vi "Connect_AMI.vi"(1 "error in":T2, 2 "Communications Config":T1={"connection ID"=refnum, "IP"="111.111.111.2", "TCP Port"=7180}) -> (0 "error out":T2)   [LabVIEW 2016]
uses:
  Instrument_Setup.vi
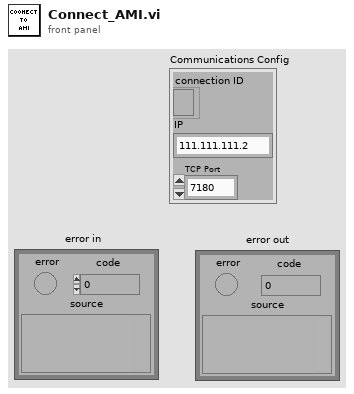
[diagram p1: front panel]
types:
  T1 = cluster{"connection ID":refnum<k5>, "IP":string, "TCP Port":i32}
  T2 = cluster{"error":bool, "code":i32, "source":string}
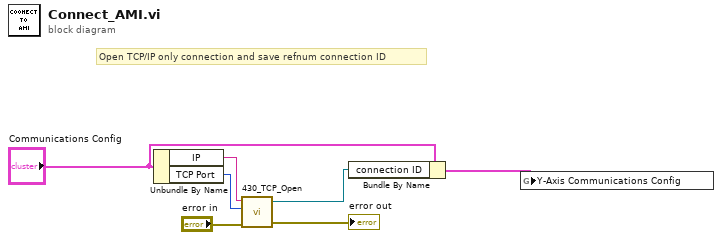
[diagram p0: block diagram]
diagram:
  # "Open TCP/IP only connection and save refnum connection ID"
  n1 = Unbundle By Name("Communications Config") -> ("IP"=w7:string, "TCP Port"=w2:i32)
  n2 = call "430_TCP_Open.vi"("IP Address"=w7, "TCP Port"=w2, "error in (no error)"="error in") -> ("connection ID"=w3:refnum<k5>, "error out"=→"error out":errorcluster)  [unwired: 3 in, 1 out]
  n3 = Bundle By Name(cluster="Communications Config", "connection ID"=w3) -> (w5:T1)
  n4 = global write "Instrument_Setup.vi" "Y-Axis Communications Config"(w5) -> ()
